vi "set DC test parameters.vi"(7 "DC Parameters":T2={"Voltage Level [V]"=1000, "Hi Limit [A]"=0.005, "Test Time [s] "=3.3, "Dwell Time [s]"=4.4, "Lo Limit [A]"=0.001, "ARC Limit [A]"=0.005, "Ramp Time [s] "=1.1, "Fall Time [s]"=2.2} {"Voltage Level [V]" min=50 max=6000 step=1 format="%.3p"; "Hi Limit [A]" min=1e-07 max=0.01 step=1e-07 format="%.2p"; "Test Time [s]" min=0.0 max=999.0 step=0.1 format="%.1p"; "Dwell Time [s]" min=0.0 max=999.0 step=0.1 format="%.1p"; "Lo Limit [A]" min=0.0 max=0.01 step=1e-06 format="%.2p"; "ARC Limit [A]" min=0.0 max=0.01 step=0.001 format="%.1p"; "Ramp Time [s]" min=0.0 max=999.0 step=0.1 format="%.1p"; "Fall Time [s]" min=0.0 max=999.0 step=0.1 format="%.1p"}, 8 "error in (no error)":errorcluster, 10 "Step":T1=1 min=1 max=99 step=1, 11 "VISA Refnum in":refnum<visa-resource-name>) -> (0 "error out":errorcluster, 3 "VISA Refnum out":refnum<visa-resource-name>)   [LabVIEW 2025]
uses:
  DC parameters--cluster.ctl
  <instrlib>/Chroma 19052/Public/Utility/Type Def/steps--numeric.ctl
  <instrlib>/Chroma 19052/Public/Utility/Type Def/AC-DC-IR modes--ring.ctl
  <instrlib>/Chroma 19052/Public/Utility/Type Def/AC-DC modes--ring.ctl
  <instrlib>/Chroma 19052/Public/Utility/Type Def/DC-IR modes--ring.ctl
  <instrlib>/Chroma 19052/Chroma 19052.lvlib
panel:
  # "DC"
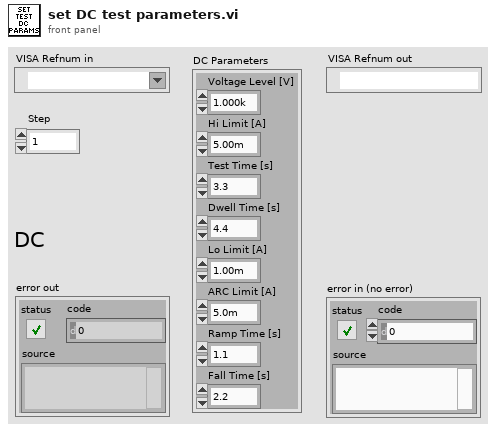
[diagram p1: front panel]
types:
  T1 = typedef "Chroma 19052.lvlib/steps--numeric.ctl" = u8
  T2 = typedef "DC parameters--cluster.ctl" = cluster{"Voltage Level [V]":u16, "Hi Limit [A]":dbl, "Test Time [s] ":dbl, "Dwell Time [s]":dbl, "Lo Limit [A]":dbl, "ARC Limit [A]":dbl, "Ramp Time [s] ":dbl, "Fall Time [s]":dbl}
  T3 = typedef "DC-IR modes--ring.ctl" = u16
  T4 = typedef "AC-DC modes--ring.ctl" = i32
  T5 = typedef "AC-DC-IR modes--ring.ctl" = u16
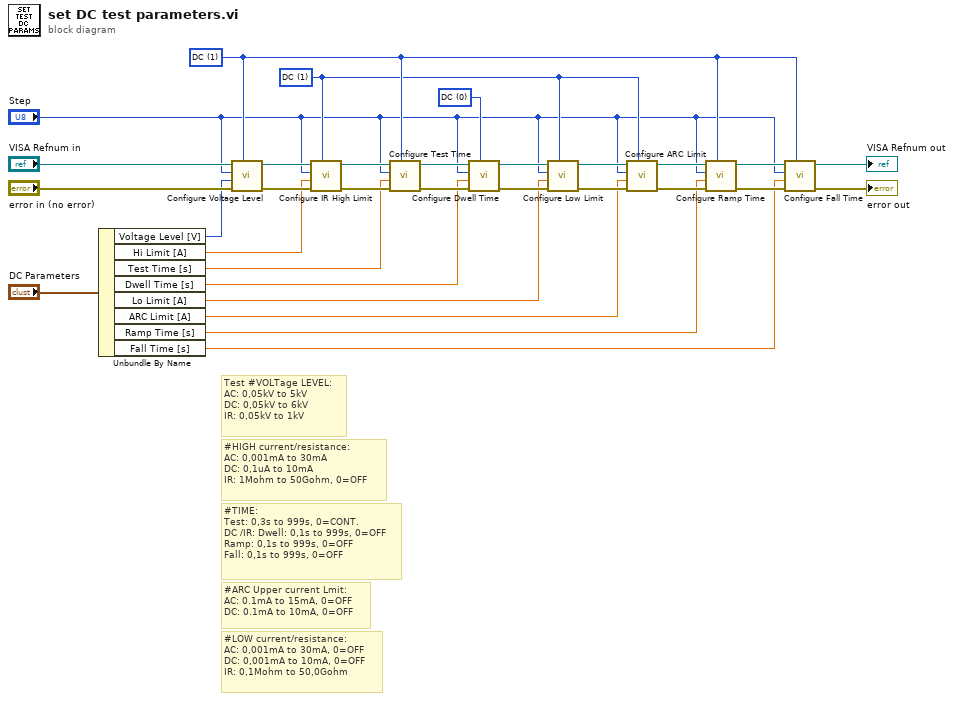
[diagram p0: block diagram]
diagram:
  w13 = T3 0 items=["DC", "IR"] ("Mode")
  w11 = T4 1 items=["AC", "DC"] ("Mode")
  w12 = T5 1 items=["AC", "DC", "IR"] ("Mode")
  # "#ARC Upper current Lmit:\nAC: 0.1mA to 15mA, 0=OFF\nDC: 0.1mA to 10mA, 0=OFF"
  # "#TIME: \nTest: 0,3s to 999s, 0=CONT. \nDC /IR: Dwell: 0,1s to 999s, 0=OFF\nRamp: 0,1s to 999s, 0=OFF\nFall: 0,1s to 999s, 0=OFF"
  # "#LOW current/resistance: \nAC: 0,001mA to 30mA, 0=OFF\nDC: 0,001mA to 10mA, 0=OFF\nIR: 0,1Mohm to 50,0Gohm"
  # "#HIGH current/resistance: \nAC: 0,001mA to 30mA\nDC: 0,1uA to 10mA\nIR: 1Mohm to 50Gohm, 0=OFF"
  # "Test #VOLTage LEVEL: \nAC: 0,05kV to 5kV\nDC: 0,05kV to 6kV\nIR: 0,05kV to 1kV"
  n1 = Unbundle By Name("DC Parameters") -> ("Voltage Level [V]"=w9:u16, "Hi Limit [A]"=w8:dbl, "Test Time [s]"=w7:dbl, "Dwell Time [s]"=w6:dbl, "Lo Limit [A]"=w1:dbl, "ARC Limit [A]"=w5:dbl, "Ramp Time [s]"=w4:dbl, "Fall Time [s]"=w3:dbl)
  n2 = call <instrlib>:"Configure Voltage Level.vi"("Mode"=w12, "error in (no error)"="error in (no error)", "Voltage Level [V]"=w9, "Step"="Step", "VISA resource name"="VISA Refnum in") -> ("error out"=w20:errorcluster, "VISA resource name out"=w17:refnum<visa-resource-name>)  [unwired: 5 in]
  n3 = call <instrlib>:"Configure IR High Limit.vi"("Mode"=w11, "error in (no error)"=w20, "Hi Limit [ohm]"=w8, "Step"="Step", "VISA resource name"=w17) -> ("error out"=w27:errorcluster, "VISA resource name out"=w28:refnum<visa-resource-name>)  [unwired: 5 in]
  n4 = call <instrlib>:"Configure Test Time.vi"("Mode"=w12, "error in (no error)"=w27, "Test Time [s]"=w7, "Step"="Step", "VISA resource name"=w28) -> ("error out"=w30:errorcluster, "VISA resource name out"=w14:refnum<visa-resource-name>)  [unwired: 5 in]
  n5 = call <instrlib>:"Configure Dwell Time.vi"("Mode"=w13, "error in (no error)"=w30, "Dwell Time [s]"=w6, "Step"="Step", "VISA resource name"=w14) -> ("error out"=w29:errorcluster, "VISA resource name out"=w31:refnum<visa-resource-name>)  [unwired: 5 in]
  n6 = call <instrlib>:"Configure Low Limit.vi"("Mode"=w11, "error in (no error)"=w29, "Lo Limit [A]"=w1, "Step"="Step", "VISA resource name"=w31) -> ("error out"=w21:errorcluster, "VISA resource name out"=w22:refnum<visa-resource-name>)  [unwired: 5 in]
  n7 = call <instrlib>:"Configure ARC Limit.vi"("Mode"=w11, "error in (no error)"=w21, "ARC Limit [A]"=w5, "Step"="Step", "VISA resource name"=w22) -> ("error out"=w23:errorcluster, "VISA resource name out"=w25:refnum<visa-resource-name>)  [unwired: 5 in]
  n8 = call <instrlib>:"Configure Ramp Time.vi"("Mode"=w12, "error in (no error)"=w23, "Ramp Time [s]"=w4, "Step"="Step", "VISA resource name"=w25) -> ("error out"=w24:errorcluster, "VISA resource name out"=w26:refnum<visa-resource-name>)  [unwired: 5 in]
  n9 = call <instrlib>:"Configure Fall Time.vi"("Mode"=w12, "error in (no error)"=w24, "Fall Time [s]"=w3, "Step"="Step", "VISA resource name"=w26) -> ("error out"=→"error out":errorcluster, "VISA resource name out"=→"VISA Refnum out":refnum<visa-resource-name>)  [unwired: 5 in]
